vi "BuildTileCode.vi"(8 "replace_color":fxp<+,3,3>, 9 "color_to_replace":fxp<+,3,3>=7.0, 10 "rotation":u8, 11 "tilenumber":u8) -> (3 "TileCode":u16)   [LabVIEW 2019, in "RT_Game.lvlib" / "Game.lvclass"]
uses:
  Game.lvclass
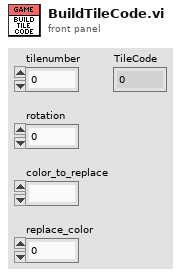
[diagram p1: front panel]
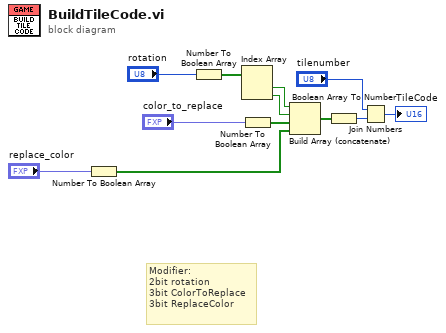
[diagram p0: block diagram]
diagram:
  # "Modifier:\n2bit rotation\n3bit ColorToReplace\n3bit ReplaceColor"
  n1 = Number To Boolean Array(number="replace_color") -> (Boolean array=w10:bool[])
  n2 = Number To Boolean Array(number="rotation") -> (Boolean array=w6:bool[])
  n3 = Index Array(array=w6) -> (element #1=w7:bool, element #2=w8:bool)  [unwired: 2 in]
  n4 = Number To Boolean Array(number="color_to_replace") -> (Boolean array=w9:bool[])
  n5 = Build Array (concatenate)(w7, w8, w9, w10) -> (w11:bool[])
  n6 = Boolean Array To Number(Boolean array=w11) -> (number=w12:u8)
  n7 = Join Numbers(hi="tilenumber", lo=w12) -> ((hi.lo)=→"TileCode":u16)
